vi "Save_RegGroups.vi"(8 "error in (no error)":errorcluster, 11 "IB_MSI in":refnum<class "IB_MSI.lvclass">) -> (0 "error out":errorcluster, 3 "IB_MSI out":refnum<class "IB_MSI.lvclass">)   [LabVIEW 2020, in "IB_MSI.lvclass"]
uses:
  <vilib>/AppBuilder/IB_Classes/MSI/IB_MSI.lvclass
  <vilib>/AppBuilder/IB_Classes/MSI/IB_MSI.lvclass/IB_MSI.ctl
  <vilib>/AppBuilder/IB_Classes/Installer/Installer.lvclass
  <vilib>/AppBuilder/IB_Classes/RegGroup/IB_RegGroup.lvclass
  e:/builds/penguin/labview/branches/2020/dev/dist/vi.lib/AppBuilder/IB_Classes/Installer/Installer.lvclass
  e:/builds/penguin/labview/branches/2020/dev/dist/vi.lib/AppBuilder/IB_Classes/MSI/IB_MSI.lvclass
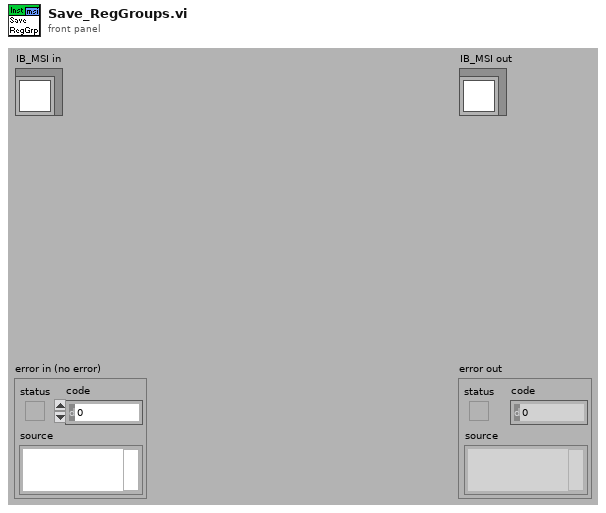
[diagram p1: front panel]
types:
  T1 = typedef "IB_Installer.ctl" = cluster{"Destination":refnum<class "IB_Destination.lvclass">[], "Source":refnum<class "IB_Source.lvclass">[], "buildObject":T2, "defaultDir":string, "platform":string, "author":string, "productName":string, "buildSpecName":string, "hide":bool, "requireLVDevSys":bool, "autoIncrement":bool, "includeError":bool, "readmeID":string, "buildLocation":path, "readmePath":path, "mediaSize":u16, "language":T3, "productVersion":T4, "preview":bool, "programmatic":bool, "progressBarEvents":T5, "userLog_Path":path, "shortcutAddresses":T7[], "EXE_Install Address":string, "EXE_Uninstall Address":string, "additional NIPaths":refnum<class "Dest_NI_NIPath.lvclass">[], "web service itemIDs":string[], "installerName":string}
  T2 = typedef "ItemRef.ctl" = u64
  T3 = typedef "CDK_sTypeDef_Languages.ctl" = u16
  T4 = typedef "CDK_sTypeDef_ProductVersion.ctl" = cluster{"Major":u8, "Minor":u8, "Update":u16}
  T5 = typedef "provcom_ProgressBar_Events.ctl" = cluster{"newJob":refnum<user-event>, "newItem":refnum<user-event>, "errorMsg":T6, "cancel":refnum<user-event>}
  T6 = typedef "mxLvBuildError.ctl" = refnum<user-event>
  T7 = typedef "CDK_sTypeDef_ShortcutAddress.ctl" = cluster{"file":string, "shortcut":string}
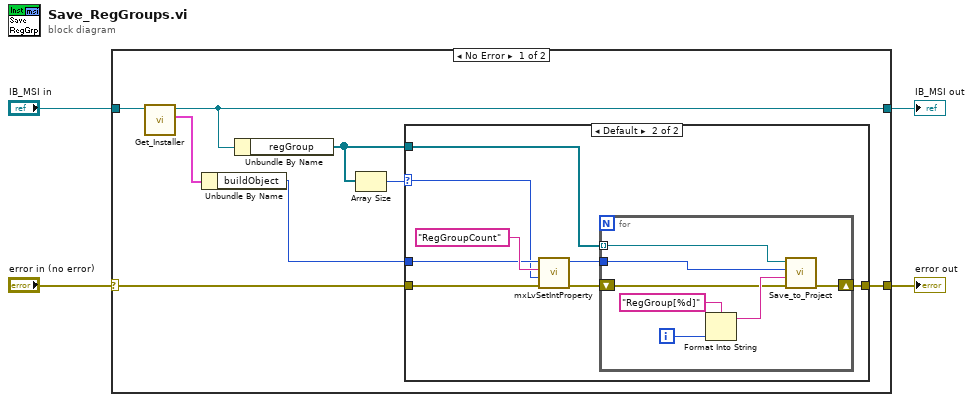
[diagram p0: block diagram]
diagram:
  n1 = case shown="No Error" "error in (no error)" {
    selector: "error in (no error)" -> [w7 w30]
    tunnel: [w6 w30] -> w3
    tunnel: [w8 w29] -> w1
    tunnel: "IB_MSI in" -> [w9 w29]
    frame No Error {
      n2 = call <vilib>:"Get_Installer.vi"("Installer in"=w9) -> ("data"=w11:T1, "Installer out"=w8:refnum<class "IB_MSI.lvclass">)  [unwired: 8 in, 1 out]
      n3 = Unbundle By Name(w11) -> ("buildObject"=w10:T2)
      n4 = Unbundle By Name(w8) -> ("regGroup"=w12:refnum<class "IB_RegGroup.lvclass">[])
      n5 = Array Size(array=w12) -> (size(s)=w5:i32)
      n6 = case shown="Default" w5 {
        selector: w5 -> [_ w14]
        tunnel: w12 -> [_ w20]
        tunnel: w10 -> [_ w17]
        tunnel: w7 -> [w13 w16]
        tunnel: [w13 w15] -> w6
        frame 0 {
        }
        frame Default {
          n7 = call <resource>:"mxLvSetIntProperty.vi"("error in"=w16, "Value (0)"=w14, "Tag"="RegGroupCount", "Item"=w17) -> ("error out"=w18:errorcluster, "Item"=w19:T2)  [unwired: 1 in, 5 out]
          n8 = for {
            tunnel: w20 -> [w25] mode=indexing
            tunnel: w19 -> [w24]
            shift-right: [w28] -> w15
            shift-left: w18 -> [w22]
            i -> [w26]
            n9 = Format Into String(format string="RegGroup[%d]", w26) -> (resulting string=w23:string)  [unwired: 2 in, 1 out]
            n10 = call <vilib>:"Save_to_Project.vi"("error in (no error)"=w22, "index in"=w23, "buildObject"=w24, "IB_RegGroup in"=w25) -> ("error out"=w28:errorcluster)  [unwired: 4 in, 3 out]
          }
        }
      }
    }
    frame Error {
    }
  }
  "error out" <- w3
  "IB_MSI out" <- w1
